vi "Create Channel.vi"(8 "error in (no error)":errorcluster, 9 "Tags":map{string, string}(c390), 10 "Channel Name":string, 11 "Nominal Streaming in":refnum<class "Nominal Streaming.lvclass">) -> (0 "error out":errorcluster, 2 "Channel":refnum<class "Channel.lvclass">, 3 "Nominal Streaming out":refnum<class "Nominal Streaming.lvclass">)   [LabVIEW 2020, in "Nominal Streaming.lvclass"]
uses:
  Nominal Streaming.lvclass
  Channel/Channel.lvclass
  Nominal Streaming.lvclass/Nominal Streaming.ctl
  target/i686-pc-windows-msvc/release/nominal_labview_ffi.dll
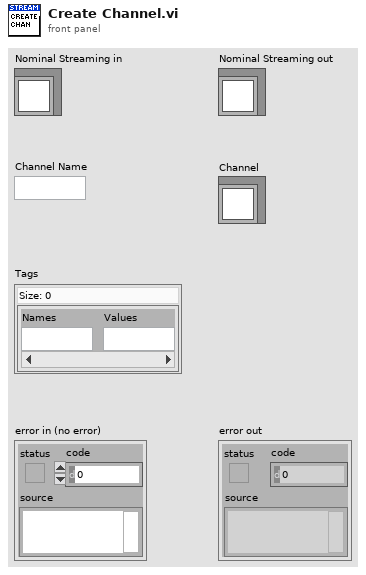
[diagram p1: front panel]
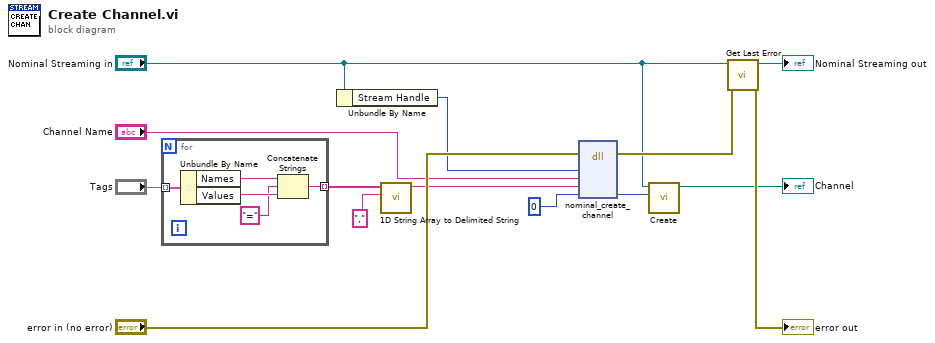
[diagram p0: block diagram]
diagram:
  n1 = for {
    tunnel: "Tags" -> [w19] mode=indexing
    tunnel: [w15] -> w10 mode=indexing
    n2 = Unbundle By Name(w19) -> ("Names"=w18:string, "Values"=w17:string)
    n3 = Concatenate Strings(w18, "=" ("string"), w17) -> (w15:string)
  }
  n4 = Unbundle By Name("Nominal Streaming in") -> ("Stream Handle"=w12:u64)
  n5 = call <vilib>:"1D String Array to Delimited String.vi"("delimiter"=",", "string array"=w10) -> ("delimited string"=w5:string)  [unwired: 9 in]
  n6 = dll-call lib="C:/code/nominal-streaming-labview-ffi/target/i686-pc-windows-msvc/release/nominal_labview_ffi.dll" fn="nominal_create_channel"(error in="error in (no error)", "stream_handle"=w12, "channel_name"="Channel Name", "tags_csv"=w5, "out_writer_handle"=u64 0) -> (error out=w7:errorcluster, "out_writer_handle"=w3:u64)  [unwired: 6 in, 1 out]
  n7 = call "Create.vi"("Channel Writer"=w3, "Nominal Streaming.lvclass"="Nominal Streaming in") -> ("Channel"=→"Channel":refnum<class "Channel.lvclass">)  [unwired: 9 in]
  n8 = call "Get Last Error.vi"("error in (no error)"=w7, "Nominal Streaming in"="Nominal Streaming in") -> ("error out"=→"error out":errorcluster, "Nominal Streaming out"=→"Nominal Streaming out":refnum<class "Nominal Streaming.lvclass">)  [unwired: 8 in]
